vi "example.vi"() -> ()   [LabVIEW 2021]
uses:
  led_globals.vi
  FSM/FSM.lvclass
panel:
  out "elapsed/remaining(ms)":cluster{"elapsed":u32, "remaining":u32}
  in  "stop":bool
  out "current state":string
  out "Counter Value":u64
  in  "button":bool
  out "LED":bool
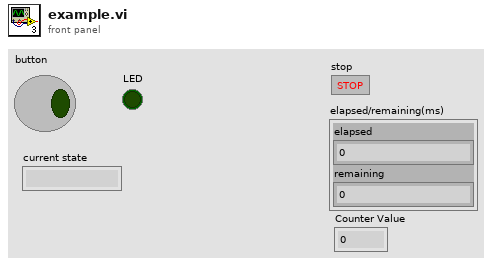
[diagram p1: front panel]
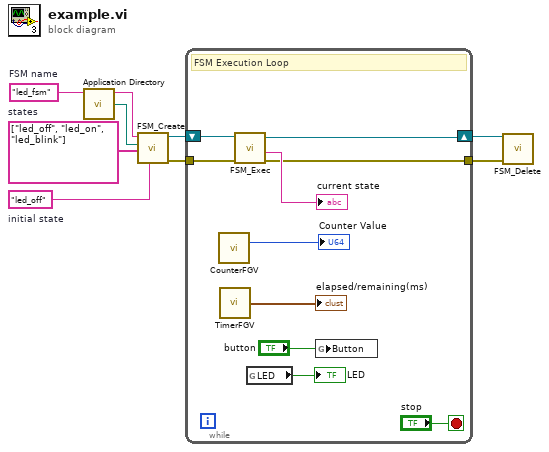
[diagram p0: block diagram]
diagram:
  w4 = "led_off"  # initial state
  w6 = string[] ["led_off", "led_on", "led_blink"]  # states
  w8 = "led_fsm"  # FSM name
  n1 = call <vilib>:"Application Directory.vi"() -> ("Application Directory"=w7:path)
  n2 = call "FSM_Create.vi"("initial state"=w4, "states"=w6, "base path"=w7, "FSM name"=w8) -> ("error out"=w1:errorcluster, "FSM"=w5:refnum<class "FSM.lvclass">)  [unwired: 6 in]
  n3 = while {
    shift-right: [w13] -> w3
    shift-left: w5 -> [w18]
    tunnel: [w11] -> w2
    tunnel: w1 -> [w9]
    stop <- "stop" stop-if-true
    # "FSM Execution Loop"
    n4 = call "CounterFGV.vi"() -> ("value"=→"Counter Value":u64)  [unwired: 14 in, 1 out]
    n5 = call "TimerFGV.vi"() -> ("elapsed/remaining(ms)"=→"elapsed/remaining(ms)":cluster{"elapsed":u32, "remaining":u32})  [unwired: 13 in, 2 out]
    n6 = call "FSM_Exec.vi"("error in (no error)"=w9, "FSM in"=w18) -> ("error out"=w11:errorcluster, "current state"=→"current state":string, "FSM out"=w13:refnum<class "FSM.lvclass">)  [unwired: 7 in]
    n7 = global read "led_globals.vi" "LED"() -> (→"LED":bool)
    n8 = global write "led_globals.vi" "Button"("button") -> ()
  }
  n9 = call "FSM_Delete.vi"("error in (no error)"=w2, "FSM"=w3) -> ()  [unwired: 9 in, 1 out]
